vi "Help.vi"   [LabVIEW 2011]
doc: "Displays a standard dialog box that prompts users to enter information, such as a user name and password.\n--------------------\n\nThis Express VI is configured as follows:\n\nMessage to Display to the User:请输入用户名和密码，登录测试软件！\nThe inputs are: \nText Entry Box: UserName\nText Entry Box: Password"
panel:
  # "HPTS Of  VNA"
  # "Developer:  EBU EE Team"
  # "Contact:  Figo Ba"
  # "E-Mail: Figo.Ba.@Luxshare-ict.com"
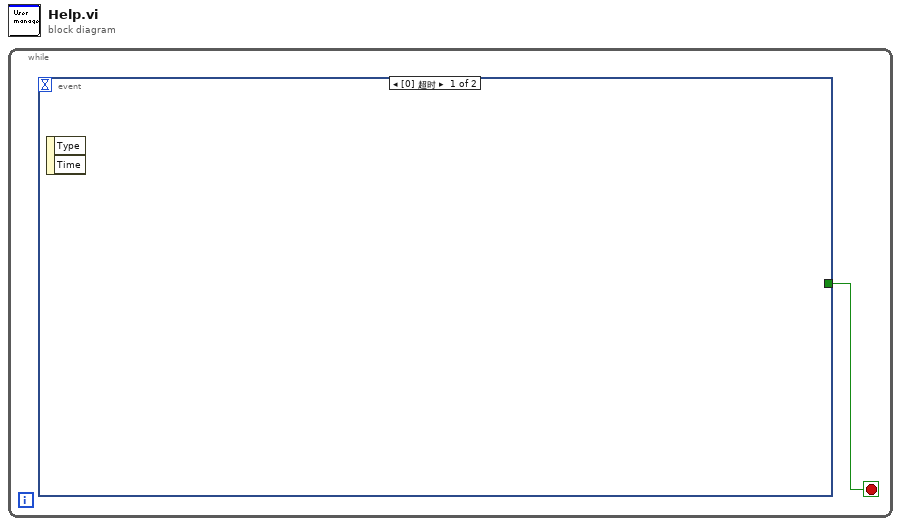
[diagram p0: block diagram]
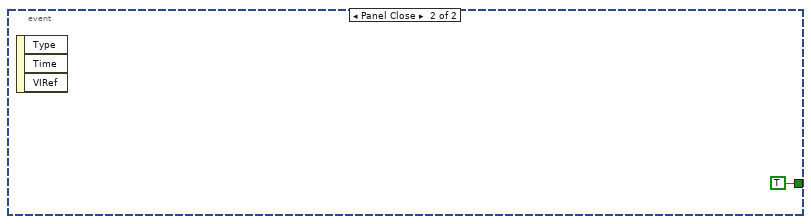
[diagram p2: hidden frame]
diagram:
  n1 = while {
    stop <- w1 stop-if-true
    n2 = event shown="[0] 超时" {
      selector: _ -> [_ _]
      dyn-events: _ -> [_ _]
      timeout: _ -> [_ _]
      tunnel: [_ TRUE ("Cancel")] -> w1
      event Timeout {
        n3 = event-data() -> ()  [unwired: 1 in, 2 out]
      }
      event Panel Close {
        n4 = event-data() -> ()  [unwired: 1 in, 3 out]
      }
    }
  }
